vi "Register for Subpanel Events.vi"(8 "error in (no error)":errorcluster, 11 "CIF_UI in":refnum<class "CIF_UI.lvclass">) -> (0 "error out":errorcluster, 3 "Event Registration Refnum":refnum<event-registration>)   [LabVIEW 2021, in "CIF_UI.lvclass"]
uses:
  CIF_UI.lvclass
  Typedef/New Connection Plugin Event Data.ctl
  CIF_UI.lvclass/CIF_UI.ctl
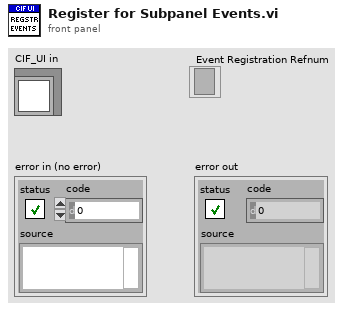
[diagram p1: front panel]
types:
  T1 = typedef "CIF_UI.lvclass/SubPanel Events.ctl" = cluster{"Clear Local Error":refnum<user-event>, "Shutdown":refnum<user-event>, "Plugin Connection":refnum<user-event>}
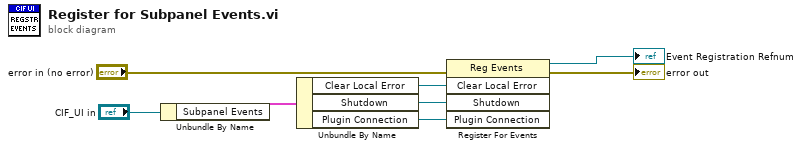
[diagram p0: block diagram]
diagram:
  n1 = Unbundle By Name("CIF_UI in") -> ("Subpanel Events"=w7:T1)
  n2 = Unbundle By Name(w7) -> ("Clear Local Error"=w6:refnum<user-event>, "Shutdown"=w5:refnum<user-event>, "Plugin Connection"=w2:refnum<user-event>)
  n3 = register-events(error in="error in (no error)", w6, w5, w2) -> (reference out=→"Event Registration Refnum":refnum<event-registration>, error out=→"error out":errorcluster)  [unwired: 1 in]
